vi "example-2.vi"(8 "error in (no error)":errorcluster) -> (0 "error out":errorcluster)   [LabVIEW 2019]
uses:
  <vilib>/numeric/Random Number (Range) DBL.vi
  e2ac90a9-f3dc-4cb2-8134-752160e7079c.vi
  f7cbbd81-eb58-4d71-bada-c91a7ecadc85.vi
  a1118f79-2200-4914-8c15-bf3ed6399d3b.vi
  f401dca3-f631-40e3-af1b-75a836bd8272.vi
  <vilib>/JDP Science/JSONtext/Make JSON Array.vi
  f7cbbd81-eb58-4d71-bada-c91a7ecadc85.vi/a5cd3052-2199-4c51-a37f-d7dc8ccacd52.vi
  f401dca3-f631-40e3-af1b-75a836bd8272.vi/4acf2560-29d2-4f78-9c39-88d1f35698bc.vi
  <vilib>/JDP Science/JSONtext/Variant to JSON Text.vi
  <vilib>/JDP Science/JSONtext/support/Format JSON Array Text.vi
  <vilib>/JDP Science/JSONtext/JSON text to Variant.vi
  <vilib>/JDP Science/JSONtext/LVClass Serializer/JSONtext LVClass Serializer.lvclass
  JSON-RPC/JSON-RPC.lvlib
panel:
  out "Data out":dbl[](array[numeric])
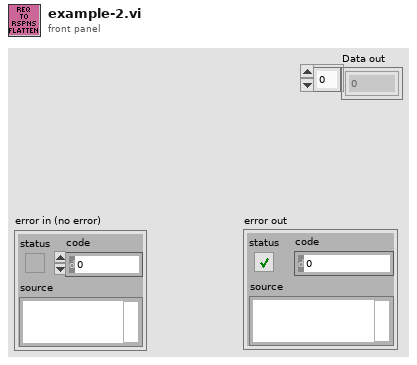
[diagram p1: front panel]
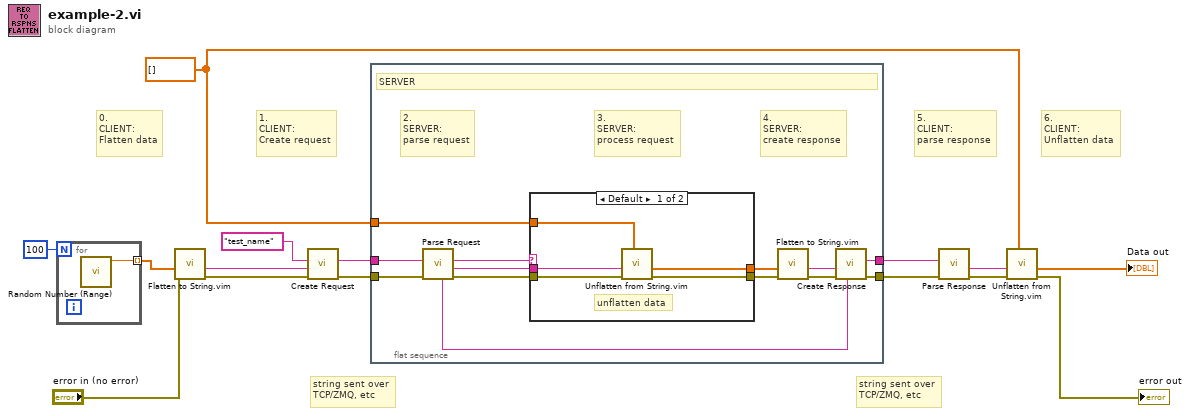
[diagram p0: block diagram]
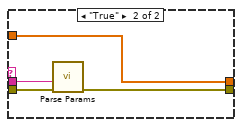
[diagram p2: hidden frame]
diagram:
  w7 = dbl[] []
  # "6.\nCLIENT:\nUnflatten data"
  # "0.\nCLIENT:\nFlatten data"
  # "string sent over\nTCP/ZMQ, etc"
  # "string sent over\nTCP/ZMQ, etc"
  # "5.\nCLIENT:\nparse response"
  # "1.\nCLIENT:\nCreate request"
  n1 = for {
    N: 100 -> [_]
    tunnel: [w16] -> w5 mode=indexing
    n2 = call-poly <vilib>:"Random Number (Range).vi"() -> ("number"=w16:dbl)  [unwired: 11 in]
  }
  n3 = call "Flatten to String.vim"("error in (no error)"="error in (no error)", "Data in"=w5) -> ("error out"=w9:errorcluster, "<JSON>"=w4:string)  [unwired: 8 in]
  n4 = call "Create Request.vi"("error in (no error)"=w9, "params"=w4, "method"="test_name") -> ("error out"=w14:errorcluster, "<JSON> Requests"=w15:string)  [unwired: 6 in, 1 out]
  n5 = flat-sequence {
    tunnel: w15 -> [w29]
    tunnel: w14 -> [w25]
    tunnel: [w24] -> w13
    tunnel: [w23] -> w12
    tunnel: w7 -> [w22]
    frame #0 {
      # "2.\nSERVER:\nparse request"
      # "3.\nSERVER:\nprocess request"
      # "4.\nSERVER:\ncreate response"
      # "SERVER"
      n6 = call "Parse Request.vi"("error in (no error)"=w25, "<JSON> Requests"=w29) -> ("error out"=w26:errorcluster, "Params"=w27:string, "Methods"=w28:string, "IDs"=w19:string)  [unwired: 6 in]
      n7 = case shown="Default" w28 {
        tunnel: w27 -> [w31 w38]
        tunnel: w26 -> [w34 w37]
        tunnel: [w33 w36] -> w20
        tunnel: w22 -> [w32 w35]
        tunnel: [w30 w35] -> w18
        frame Default {
          # "unflatten data"
          n8 = call "Unflatten from String.vim"("type"=w32, "error in (no error)"=w34, "<JSON>"=w31) -> ("error out"=w33:errorcluster, "Data out"=w30:dbl[])  [unwired: 7 in]
        }
        frame "True" {
          n9 = call "Parse Params.vi"("error in (no error)"=w37, "<JSON> Params"=w38) -> ("error out"=w36:errorcluster)  [unwired: 7 in, 2 out]
        }
      }
      n10 = call "Flatten to String.vim"("error in (no error)"=w20, "Data in"=w18) -> ("error out"=w21:errorcluster, "<JSON>"=w17:string)  [unwired: 8 in]
      n11 = call "Create Response.vi"("id"=w19, "error in (no error)"=w21, "result"=w17) -> ("error out"=w23:errorcluster, "<JSON> Response"=w24:string)  [unwired: 7 in]
    }
  }
  n12 = call "Parse Response.vi"("error in (no error)"=w12, "<JSON> Response"=w13) -> ("error out"=w8:errorcluster, "results"=w3:string)  [unwired: 7 in, 1 out]
  n13 = call "Unflatten from String.vim"("type"=w7, "error in (no error)"=w8, "<JSON>"=w3) -> ("error out"=→"error out":errorcluster, "Data out"=→"Data out":dbl[])  [unwired: 7 in]
